vi "Convert all SVGs to PNGs.vi"   [LabVIEW 2023, in "VILab.lvlib"]
uses:
  VILab.lvlib
  <userlib>/_OpenG.lib/file/file.llb/openg_file.lvlib
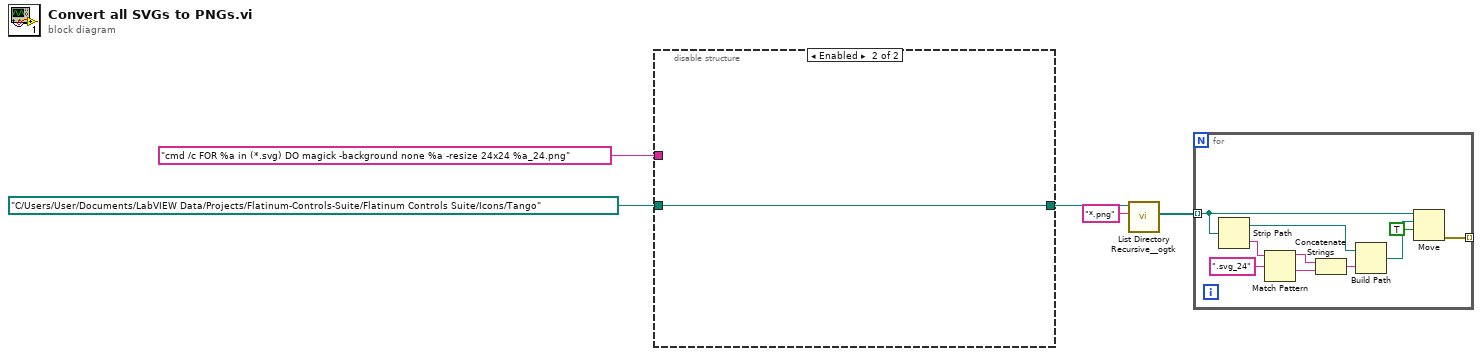
[diagram p0: block diagram]
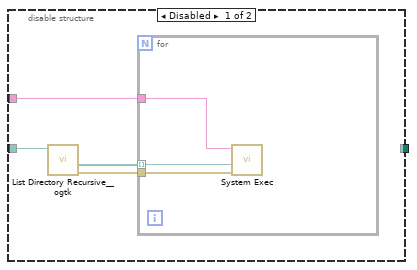
[diagram p2: hidden frame]
diagram:
  n1 = disable-structure shown="Enabled" {
    disable-tunnel: path "C:/Users/User/Documents/LabVIEW Data/Projects/Flatinum-Controls-Suite/Flatinum Controls Suite/Icons/Tango" ("Path") -> [w8 w13]
    disable-tunnel: "cmd /c FOR %a in (*.svg) DO magick -background none %a -resize 24x24 %a_24.png" -> [w7 _]
    disable-tunnel: [_ w13] -> w3
    frame Disabled {
      n2 = call <userlib>:"List Directory Recursive__ogtk.vi"("Path"=w8) -> ("error out"=w9:errorcluster, "dir paths"=w6:path[])  [unwired: 7 in, 2 out]
      n3 = for {
        tunnel: w9 -> [w12]
        tunnel: w7 -> [w11]
        tunnel: w6 -> [w10] mode=indexing
        n4 = call <vilib>:"System Exec.vi"("error in (no error)"=w12, "working directory"=w10, "command line"=w11) -> ()  [unwired: 5 in, 4 out]
      }
    }
    frame Enabled {
    }
  }
  n5 = call <userlib>:"List Directory Recursive__ogtk.vi"("pattern"="*.png", "Path"=w3) -> ("file paths"=w1:path[])  [unwired: 6 in, 3 out]
  n6 = for {
    tunnel: w1 -> [w22] mode=indexing
    tunnel: [w15] -> _ mode=indexing
    n7 = Strip Path(path=w22) -> (stripped path=w18:path, name=w21:string)
    n8 = Match Pattern(string=w21, regular expression=".svg_24") -> (before substring=w20:string, after substring=w19:string)  [unwired: 1 in, 2 out]
    n9 = Concatenate Strings(w20, w19) -> (w17:string)
    n10 = Build Path(base path=w18, name or relative path=w17) -> (appended path=w16:path)
    n11 = Move(source path=w22, 9:TRUE ("overwrite (F)"), 10:w16) -> (error out=w15:errorcluster)  [unwired: 2 in, 2 out]
  }
